vi "Multiplicacion.vi"(8 "error in (no error)":errorcluster, 11 "Calculadora in":refnum<class "Calculadora.lvclass">) -> (0 "error out":errorcluster, 3 "Calculadora out":refnum<class "Calculadora.lvclass">)   [LabVIEW 2020, in "Calculadora.lvlib" / "Calculadora.lvclass"]
uses:
  Calculadora.lvclass
  Calculadora.lvclass/Calculadora.ctl
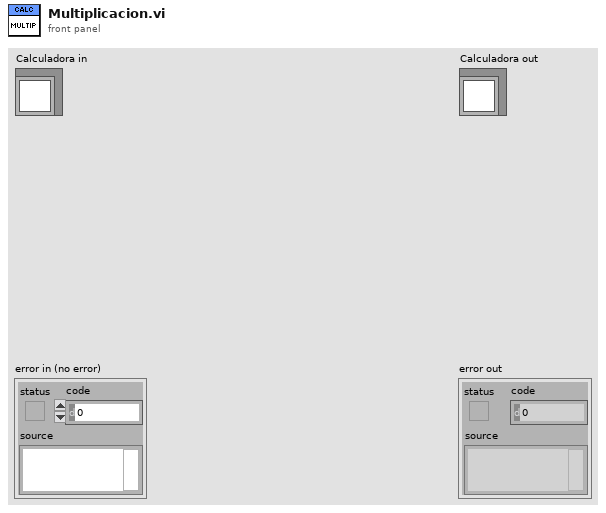
[diagram p1: front panel]
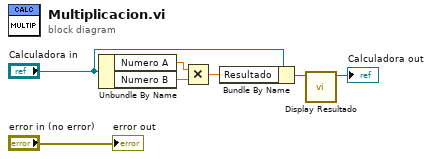
[diagram p0: block diagram]
diagram:
  n1 = Unbundle By Name("Calculadora in") -> ("Numero A"=w6:dbl, "Numero B"=w5:dbl)
  n2 = Multiply(x=w6, y=w5) -> (x*y=w4:dbl)
  n3 = Bundle By Name(cluster="Calculadora in", "Resultado"=w4) -> (w2:refnum<class "Calculadora.lvclass">)
  n4 = call "Display Resultado.vi"("Calculadora in"=w2) -> ("Calculadora out"=→"Calculadora out":refnum<class "Calculadora.lvclass">)  [unwired: 9 in, 1 out]
  "error out" <- "error in (no error)"
